vi "TranslatorBooster Build VI Outputs.vi"(8 "error in (no error)":errorcluster, 9 "Pointer?":bool, 10 "Output type":string, 11 "VI in":refnum<vi>) -> (0 "error out":errorcluster, 2 "OutputType abbr.":string, 3 "VI out":refnum<vi>)   [LabVIEW 2014, in "Complex Numbers.lvlib"]
uses:
  <vilib>/Aledyne-TSXperts/Arduino Compatible Compiler for LabVIEW/addons/Complex Numbers/Complex Numbers.lvlib
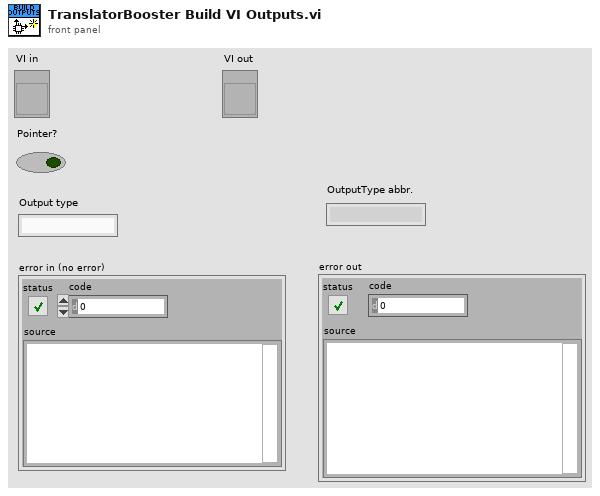
[diagram p1: front panel]
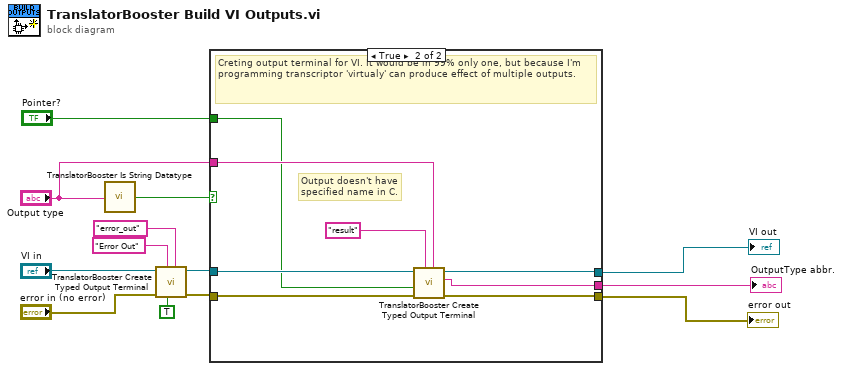
[diagram p0: block diagram]
diagram:
  n1 = call <vilib>:"TranslatorBooster Is String Datatype.vi"("String token"="Output type") -> ("Is datatype?"=w9:bool)
  n2 = call <vilib>:"TranslatorBooster Create Typed Output Terminal.vi"("Param type"="error_out", "Reset?"=TRUE, "Input name"="Error Out", "Error In"="error in (no error)", "parent VI"="VI in") -> ("Error Out"=w4:errorcluster, "parent VI out"=w5:refnum<vi>)  [unwired: 4 in, 1 out]
  n3 = case shown="True" w9 {
    tunnel: w5 -> [w14 w23]
    tunnel: [w14 w22] -> w12
    tunnel: w4 -> [w15 w20]
    tunnel: [w15 w21] -> w13
    tunnel: "Output type" -> [_ w19]
    tunnel: [_ w16] -> w10
    tunnel: "Pointer?" -> [_ w17]
    frame False {
    }
    frame True {
      # "Output doesn't have\nspecified name in C."
      # "Creting output terminal for VI. It would be in 99% only one, but because I'm\nprogramming transcriptor 'virtualy' can produce effect of multiple outputs."
      n4 = call <vilib>:"TranslatorBooster Create Typed Output Terminal.vi"("Param type"=w19, "Input name"="result" ("f"), "Error In"=w20, "Pointer?"=w17, "parent VI"=w23) -> ("Error Out"=w21:errorcluster, "OutputType abbr."=w16:string, "parent VI out"=w22:refnum<vi>)  [unwired: 4 in]
    }
  }
  "error out" <- w13
  "VI out" <- w12
  "OutputType abbr." <- w10
